vi "Measure-SM1000-conversion.vi"(8 "error in (no error)":errorcluster, 9 "Device index":i32, 10 "File path":path, 11 "SM1000-control in":T2) -> (0 "error out":errorcluster, 2 "Position data":i16[][](array[numeric]), 3 "SM1000-control out":T2)   [LabVIEW 2013, in "HardwareCharacterization.lvlib" / "HC-SM1000.lvclass"]
uses:
  HC-SM1000.lvclass
  Object-reference.ctl
  Device-identification.ctl
  EC1000_DOTNET/getBroadcastData-status.vi
panel:
  out "Identifier":T1
  out "Graph":i16[][](graph)
  in  "Start job":bool
  out "Job busy":bool
  in  "Stop":bool
  out "Elapsed time":dbl caption="Elapsed time [ms]" format="%.2f"
  out "Initialized":bool
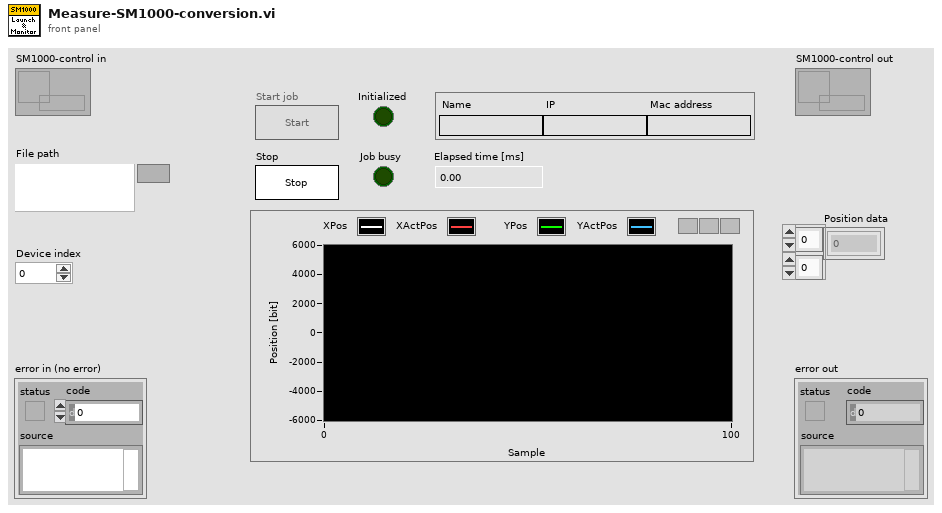
[diagram p1: front panel]
types:
  T1 = typedef "HardwareCharacterization.lvlib/HC-SM1000.lvclass/Device-identification.ctl" = cluster{"Name":string, "IP":string, "Mac address":string}
  T2 = typedef "HardwareCharacterization.lvlib/HC-SM1000.lvclass/Object-reference.ctl" = refnum<data-value>
  T3 = enum8{"Enabled", "Disabled", "Disabled and Grayed Out"}
  T4 = typedef "HardwareCharacterization.lvlib/HC-SM1000.lvclass/Status-information.ctl" = cluster{"XPosAck":bool, "YPosAck":bool, "XPos":i16, "YPos":i16, "XActPos":i16, "YActPos":i16, "XTemp":bool, "YTemp":bool, "ContrlTemp":i16, "XStatus":bool[], "YStatus":bool[], "XPower":bool, "YPower":bool, "Interlock":bool[], "CurrentDIO":bool[], "JobMarker":u16, "JobDataCntr":u32}
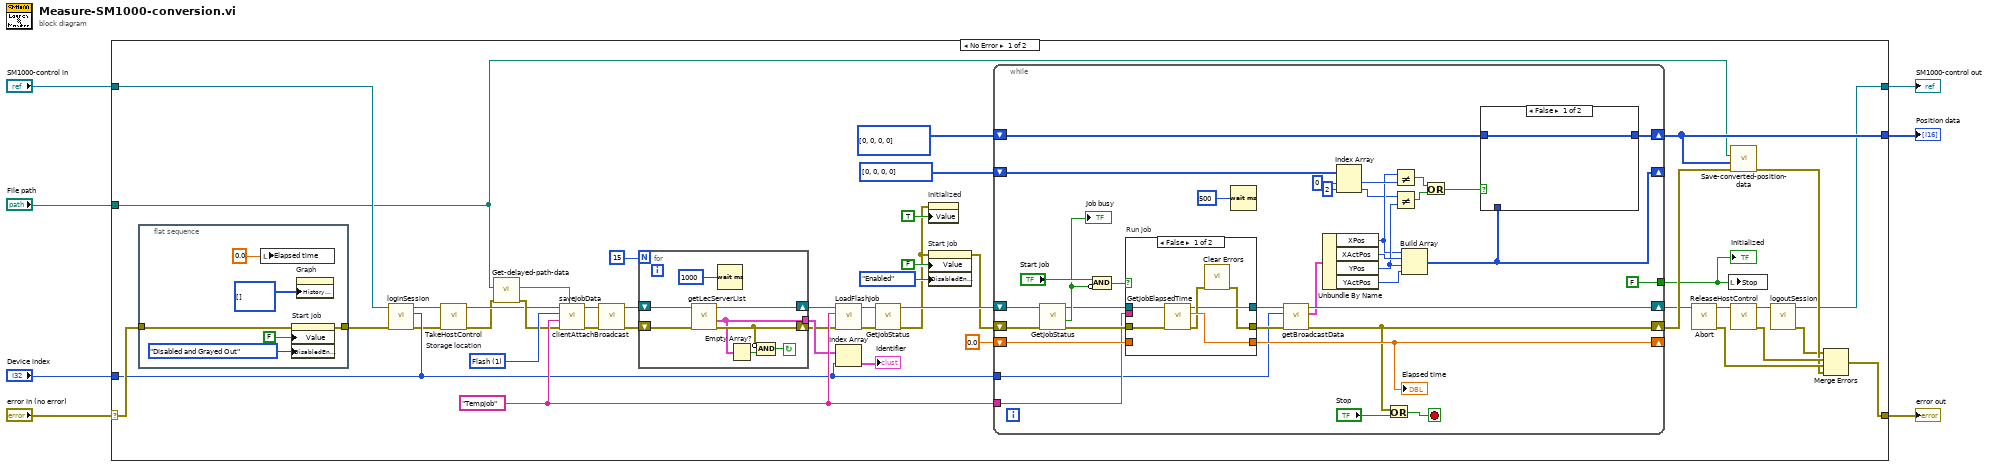
[diagram p0: block diagram]
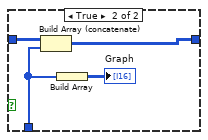
[diagram p2: hidden frame]
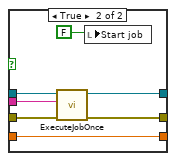
[diagram p3: hidden frame]
diagram:
  n1 = case shown="No Error" "error in (no error)" {
    selector: "error in (no error)" -> [w19 w121]
    tunnel: [w40 w121] -> w6
    tunnel: [w32 w120] -> w4
    tunnel: "SM1000-control in" -> [w45 w120]
    tunnel: "File path" -> [w34 _]
    tunnel: "Device index" -> [w17 _]
    tunnel: [w37 _] -> w1
    frame No Error {
      w50 = u16 1 items=["Flash"=1, "USB"=2]  # Storage location
      w47 = "Tempjob"
      n2 = flat-sequence {
        tunnel: [w56] -> w20
        tunnel: w19 -> [w54]
        frame #0 {
          n3 = local write "Elapsed time"(0.0 ("Elapsed time")) -> ()
          n4 = property on="Start job" class="Bool (strict)"(error in=w54, "Value"=FALSE, "DisabledEnum"=T3."Disabled and Grayed Out" ("Disabled")) -> (error out=w56:errorcluster)  [unwired: 1 in, 1 out]
          n5 = property on="Graph" class="WFChart (strict)"("History Data"=i16[][] []) -> ()  [unwired: 2 in, 2 out]
        }
      }
      n6 = call "loginSession.vi"("error in (no error)"=w20, "Device index"=w17, "SM1000-control in"=w45) -> ("error out"=w12:errorcluster, "SM1000-control out"=w13:T2)  [unwired: 7 in]
      n7 = call "TakeHostControl.vi"("error in (no error)"=w12, "SM1000-control in"=w13) -> ("error out"=w10:errorcluster, "SM1000-control out"=w11:T2)  [unwired: 8 in]
      n8 = call "Get-delayed-path-data.vi"("error in (no error)"=w10, "File path"=w34) -> ("error out"=w39:errorcluster, "Formatted contents"=w38:string)  [unwired: 8 in]
      n9 = call "saveJobData.vi"("Job data xml"=w38, "error in (no error)"=w39, "File name wo extension"=w47, "Storage location"=w50, "SM1000-control in"=w11) -> ("error out"=w28:errorcluster, "SM1000-control out"=w29:T2)  [unwired: 5 in]
      n10 = call "clientAttachBroadcast.vi"("error in (no error)"=w28, "SM1000-control in"=w29) -> ("error out"=w26:errorcluster, "SM1000-control out"=w27:T2)  [unwired: 7 in, 1 out]
      n11 = for {
        N: 15 -> [_]
        shift-right: [w64] -> w8
        shift-left: w27 -> [w66]
        shift-right: [w61] -> w9
        shift-left: w26 -> [w65]
        tunnel: [w59] -> w18
        stop <- w60 continue-if-true
        n12 = call "getLecServerList.vi"("error in (no error)"=w65, "SM1000-control in"=w66) -> ("error out"=w61:errorcluster, "Device identifiers"=w59:T1[], "SM1000-control out"=w64:T2)  [unwired: 6 in, 1 out]
        n13 = Wait (ms)(milliseconds to wait=u32 1000) -> ()  [unwired: 1 out]
        n14 = Empty Array?(array=w59) -> (empty?=w62:bool)
        n15 = Compound Arithmetic op=AND(invert w61, w62) -> (w60:bool)
      }
      n16 = call "LoadFlashJob.vi"("error in (no error)"=w9, "Job name wo extension"=w47, "SM1000-control in"=w8) -> ("error out"=w52:errorcluster, "SM1000-control out"=w51:T2)  [unwired: 7 in]
      n17 = Index Array(array=w18, index=w17) -> (element=→"Identifier":T1)
      n18 = call "GetJobStatus.vi"("error in (no error)"=w52, "SM1000-control in"=w51) -> ("error out"=w14:errorcluster, "SM1000-control out"=w49:T2)  [unwired: 7 in, 1 out]
      n19 = property on="Initialized" class="Bool (strict)"(error in=w14, "Value"=TRUE ("Initialized")) -> ()  [unwired: 1 in, 2 out]
      n20 = property on="Start job" class="Bool (strict)"(error in=w14, "Value"=FALSE, "DisabledEnum"=T3."Enabled" ("Disabled")) -> (error out=w24:errorcluster)  [unwired: 1 in, 1 out]
      n21 = while {
        shift-right: [w87] -> w36
        shift-left: w24 -> [w100]
        shift-right: [w85] -> w30
        shift-left: w49 -> [w101]
        shift-right: [w91] -> _
        shift-left: 0.0 ("Elapsed time") -> [w92]
        tunnel: w47 -> [w90]
        tunnel: [FALSE] -> w22
        tunnel: w17 -> [w83]
        shift-right: [w78] -> w37
        shift-left: i16[][] [[0, 0, 0, 0]] ("appended array") -> [w77]
        shift-right: [w79] -> _
        shift-left: i16[] [0, 0, 0, 0] ("appended array") -> [w76]
        stop <- w95 stop-if-true
        n22 = call "GetJobStatus.vi"("error in (no error)"=w100, "SM1000-control in"=w101) -> ("error out"=w94:errorcluster, "Busy?"=w97:bool, "SM1000-control out"=w93:T2)  [unwired: 7 in]
        "Job busy" <- w97
        n23 = Compound Arithmetic op=AND("Start job", invert w97) -> (w98:bool)
        n24 = case "Run job" shown="False" w98 {
          tunnel: w94 -> [w110 w116]
          tunnel: [w107 w115] -> w88
          tunnel: [w108 w114] -> w86
          tunnel: w93 -> [w112 w117]
          tunnel: [w111 w119] -> w91
          tunnel: w92 -> [_ w119]
          tunnel: w90 -> [_ w118]
          frame False {
            n25 = call "GetJobElapsedTime.vi"("error in (no error)"=w110, "SM1000-control in"=w112) -> ("error out"=w109:errorcluster, "Elapsed time"=w111:dbl, "SM1000-control out"=w108:T2)  [unwired: 7 in]
            n26 = call <vilib>:"Clear Errors.vi"("error in (no error)"=w109) -> ("error out"=w107:errorcluster)  [unwired: 6 in]
          }
          frame True {
            n27 = call "ExecuteJobOnce.vi"("error in (no error)"=w116, "Job name wo extension"=w118, "SM1000-control in"=w117) -> ("error out"=w115:errorcluster, "SM1000-control out"=w114:T2)  [unwired: 7 in]
            n28 = local write "Start job"(FALSE) -> ()
          }
        }
        "Elapsed time" <- w91
        n29 = Wait (ms)(milliseconds to wait=u32 500) -> ()  [unwired: 1 out]
        n30 = call-poly "getBroadcastData.vi"("error in (no error)"=w88, "Device index"=w83, "SM1000-control in"=w86) -> ("error out"=w87:errorcluster, "Status information"=w80:T4, "SM1000-control out"=w85:T2)  [unwired: 6 in]
        n31 = Unbundle By Name(w80) -> ("XPos"=w73:i16, "XActPos"=w82:i16, "YPos"=w75:i16, "YActPos"=w81:i16)
        n32 = Index Array(array=w76, index #1=0 ("index"), index #2=2 ("index")) -> (element #1=w74:i16, element #2=w69:i16)
        n33 = Or(x=w87, y="Stop") -> (x .or. y?=w95:bool)
        n34 = Not Equal?(x=w73, y=w74) -> (x != y?=w71:bool)
        n35 = Not Equal?(x=w69, y=w75) -> (x != y?=w72:bool)
        n36 = Build Array(w73, w82, w75, w81) -> (w79:i16[])
        n37 = Or(x=w71, y=w72) -> (x .or. y?=w70:bool)
        n38 = case shown="False" w70 {
          tunnel: w77 -> [w102 w106]
          tunnel: w79 -> [_ w103]
          tunnel: [w102 w105] -> w78
          frame False {
          }
          frame True {
            n39 = Build Array (concatenate)(w106, w103) -> (w105:i16[][])
            n40 = Build Array(w103) -> (→"Graph":i16[][])
          }
        }
      }
      "Initialized" <- w22
      n41 = call "Abort.vi"("SM1000-control in"=w30) -> ("error out"=w41:errorcluster, "SM1000-control out"=w46:T2)  [unwired: 9 in]
      n42 = local write "Stop"(w22) -> ()
      n43 = call "Save-converted-position-data.vi"("error in (no error)"=w36, "Position data"=w37, "File path"=w34) -> ("error out"=w35:errorcluster)  [unwired: 8 in]
      n44 = call "ReleaseHostControl.vi"("SM1000-control in"=w46) -> ("error out"=w42:errorcluster, "SM1000-control out"=w33:T2)  [unwired: 9 in]
      n45 = call "logoutSession.vi"("SM1000-control in"=w33) -> ("error out"=w31:errorcluster, "SM1000-control out"=w32:T2)  [unwired: 9 in]
      n46 = Merge Errors(w31, w42, w41, w35) -> (w40:errorcluster)
    }
    frame Error {
    }
  }
  "error out" <- w6
  "SM1000-control out" <- w4
  "Position data" <- w1
